vi "SV Chirp Waveform.vi"(0 "frequency range":T1={"start frequency [Hz]"=10.0, "stop frequency [Hz]"=10000.0} {"stop frequency [Hz]" format="%.2f"; "start frequency [Hz]" format="%.2f"}, 1 "reset signal (F)":bool, 5 "chirp duration [s]":dbl=-1.0, 7 "amplitude":dbl=1.0 format="%.2f", 9 "phase in [deg]":dbl format="%.2f", 11 "error in (no error)":errorcluster, 12 "sampling info":cluster{"Fs":dbl, "#s":u32}={"Fs"=51200.0, "#s"=1024} {"Fs" format="%.2p"}, 13 "frequency spacing":enum16{"Linear", "Logarithmic"}(ring)) -> (4 "chirp signal":waveform(dbl), 10 "phase out [deg]":dbl=nan, 15 "error out":errorcluster)   [LabVIEW 2017, in "SoundVib_Generation.lvlib"]
doc: "Generates a continuous chirp waveform. You can use the generated chirp waveform to perform continuous swept-sine measurements."
uses:
  <vilib>/addons/_NISVFA/_Generation/SoundVib_Generation.lvlib
  <vilib>/addons/_NISVFA/_Generation/subVIs/sv_Chirp Settings.ctl
  <vilib>/Analysis/1siggen.llb/Ramp Pattern.vi
  <vilib>/Analysis/1siggen.llb/Ramp Pattern by Samples.vi
  <vilib>/measure/NI_MABase.lvlib
panel:
  in  "waveform_empty":waveform(dbl)={"t0"=timestamp(0 s since 1904-01-01), "dt"=0.0, "Y"=[]}
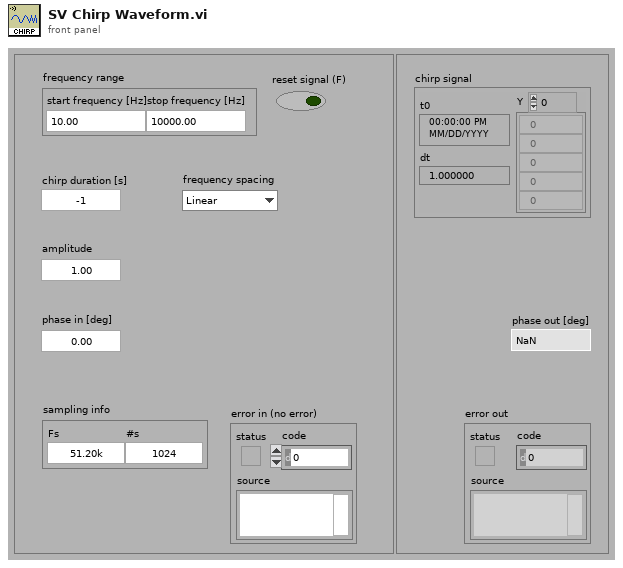
[diagram p1: front panel]
types:
  T1 = cluster{"start frequency [Hz]":dbl, "stop frequency [Hz]":dbl}
  T2 = typedef "SoundVib_Generation.lvlib/sv_Chirp Settings.ctl" = cluster{"amplitude":dbl, "frequency range":cluster{"start (Hz)":dbl, "stop (Hz)":dbl, "frequency spacing":enum16{"Linear", "Logarithmic"}}, "sampling info":cluster{"Fs":dbl, "chirp duration [s]":dbl}, "initial states":cluster{"frequency [Hz]":dbl, "phase [rad]":dbl, "elapsed time [s]":dbl}, "frequency slope":dbl, "maximum harmonic":i32, "prefix len [samples]":cluster{"integer":u32, "fractional":dbl}}
  T3 = cluster{"frequency [Hz]":dbl, "phase [rad]":dbl, "elapsed time [s]":dbl}
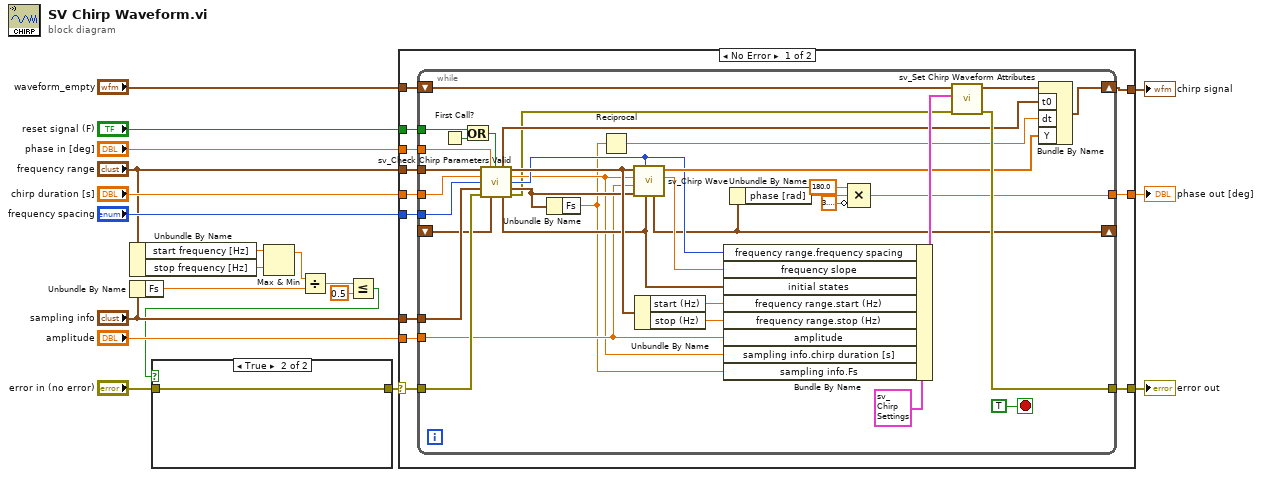
[diagram p0: block diagram]
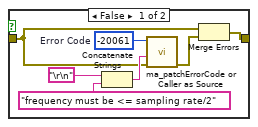
[diagram p2: hidden frame]
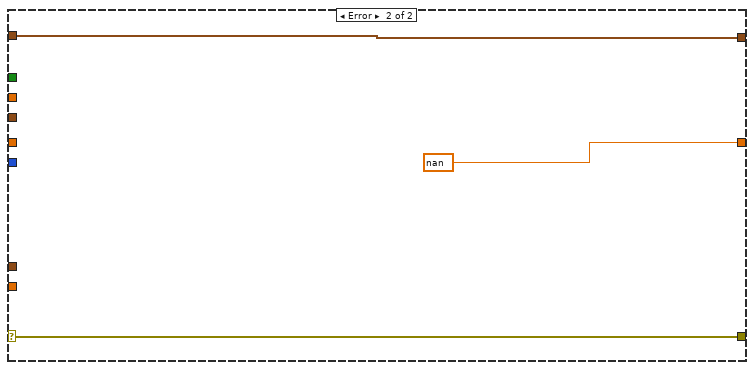
[diagram p3: hidden frame]
diagram:
  n1 = Unbundle By Name("frequency range") -> ("start frequency [Hz]"=w9:dbl, "stop frequency [Hz]"=w8:dbl)
  n2 = Unbundle By Name("sampling info") -> ("Fs"=w7:dbl)
  n3 = Max & Min(x=w9, y=w8) -> (max(x,y)=w1:dbl)  [unwired: 1 out]
  n4 = Divide(x=w1, y=w7) -> (x/y=w6:dbl)
  n5 = Less Or Equal?(x=w6, y=0.5) -> (x <= y?=w2:bool)
  n6 = case shown="True" w2 {
    tunnel: [w21 w28] -> w4
    tunnel: "error in (no error)" -> [w23 w28]
    frame False {
      w24 = -20061  # Error Code
      n7 = Concatenate Strings("\r\n", "frequency must be <= sampling rate/2" ("freq error message")) -> (w27:string)
      n8 = call <vilib>:"ma_patchErrorCode or Caller as Source.vi"("error in (no error)"=w23, "string to append to source"=w27, "error code"=w24) -> ("error out"=w22:errorcluster)  [unwired: 8 in]
      n9 = Merge Errors(w23, w22) -> (w21:errorcluster)
    }
    frame True {
    }
  }
  n10 = case shown="No Error" w4 {
    selector: w4 -> [w40 w79]
    tunnel: "sampling info" -> [w37 _]
    tunnel: "frequency range" -> [w36 _]
    tunnel: "chirp duration [s]" -> [w33 _]
    tunnel: "amplitude" -> [w35 _]
    tunnel: [w38 w79] -> w18
    tunnel: [w39 w77] -> w17
    tunnel: "reset signal (F)" -> [w29 _]
    tunnel: "frequency spacing" -> [w32 _]
    tunnel: "phase in [deg]" -> [w31 _]
    tunnel: [w34 nan] -> w13
    tunnel: "waveform_empty" -> [w30 w77]
    frame No Error {
      n11 = while {
        tunnel: w40 -> [w76]
        tunnel: [w74] -> w38
        tunnel: w37 -> [w65]
        tunnel: w36 -> [w73]
        tunnel: w35 -> [w55]
        tunnel: [w42] -> w34
        tunnel: w33 -> [w71]
        tunnel: w32 -> [w66]
        tunnel: w31 -> [w58]
        shift-right: [w46] -> _
        shift-left: _ -> [w64]
        shift-right: [w69] -> w39
        shift-left: w30 -> [w68]
        tunnel: w29 -> [w50]
        stop <- TRUE stop-if-true
        n12 = First Call?() -> (First Call?: T/F=w52:bool)
        n13 = Or(x=w50, y=w52) -> (x .or. y?=w51:bool)
        n14 = call <vilib>:"sv_Check Chirp Parameters Valid.vi"("frequency range"=w73, "phase in [deg]"=w58, "reset signal (F)"=w51, "chirp duration [s]"=w71, "frequency spacing"=w66, "sampling info"=w65, "error in (no error)"=w76, "state in"=w64) -> ("t0"=w53:timestamp, "frequency range out"=w63:cluster{"start (Hz)":dbl, "stop (Hz)":dbl}, "chirp duration [s] out"=w48:dbl, "frequency spacing out"=w49:enum16{"Linear", "Logarithmic"}, "sampling info out"=w56:cluster{"Fs":dbl, "#s":u32}, "state out"=w60:T3, "error out"=w41:errorcluster)  [unwired: 1 in]
        n15 = Unbundle By Name(w56) -> ("Fs"=w47:dbl)
        n16 = Reciprocal(x=w47) -> (1/x=w54:dbl)
        n17 = call <vilib>:"sv_Chirp Wave.vi"("state in"=w60, "frequency spacing"=w49, "sampling info"=w56, "amplitude"=w55, "chirp duration [s]"=w48, "frequency range"=w63) -> ("frequency slope"=w59:dbl, "chirp wave"=w57:dbl[], "state out"=w46:T3)  [unwired: 3 in]
        n18 = Unbundle By Name(w63) -> ("start (Hz)"=w62:dbl, "stop (Hz)"=w61:dbl)
        n19 = Bundle By Name(cluster=T2 {"amplitude"=1.0, "frequency range"={"start (Hz)"=20.0, "stop (Hz)"=20000.0, "frequency spacing"=enum."Logarithmic"}, "sampling info"={"Fs"=50000.0, "chirp duration [s]"=3.0}, "initial states"={"frequency [Hz]"=20.0, "phase [rad]"=0.0, "elapsed time [s]"=0.0}, "frequency slope"=0.0, "maximum harmonic"=3, "prefix len [samples]"={"integer"=0, "fractional"=0.0}} ("chirp settings"), "frequency range.frequency spacing"=w49, "frequency slope"=w59, "initial states"=w60, "frequency range.start (Hz)"=w62, "frequency range.stop (Hz)"=w61, "amplitude"=w55, "sampling info.chirp duration [s]"=w48, "sampling info.Fs"=w47) -> (w72:T2)
        n20 = Unbundle By Name(w46) -> ("phase [rad]"=w45:dbl)
        n21 = Compound Arithmetic op=MULTIPLY(180.0 ("value"), w45, invert 3.141592653589793) -> (w42:dbl)
        n22 = call <vilib>:"sv_Set Chirp Waveform Attributes.vi"("error in (no error)"=w41, "chirp settings"=w72, "chirp signal"=w68) -> ("error out"=w74:errorcluster, "chirp signal out"=w67:waveform(dbl))  [unwired: 7 in]
        n23 = Bundle By Name(cluster=w67, "t0"=w53, "dt"=w54, "Y"=w57) -> (w69:waveform(dbl))
      }
    }
    frame Error {
    }
  }
  "error out" <- w18
  "chirp signal" <- w17
  "phase out [deg]" <- w13
